vi "flush_trigger_queue.vi"(8 "error in (no error)":errorcluster, 11 "GenericToplevelComponent in":refnum<class "GenericToplevelComponent.lvclass">) -> (0 "error out":errorcluster, 3 "GenericToplevelComponent out":refnum<class "GenericToplevelComponent.lvclass">)   [LabVIEW 2010, in "GenericToplevelComponent.lvclass"]
uses:
  GenericToplevelComponent.lvclass
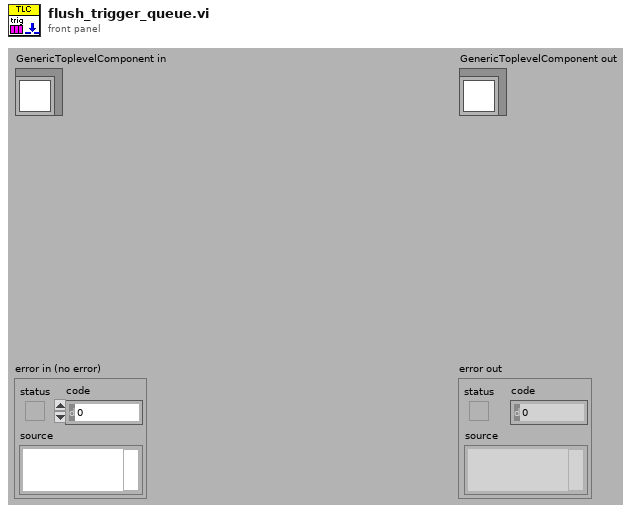
[diagram p1: front panel]
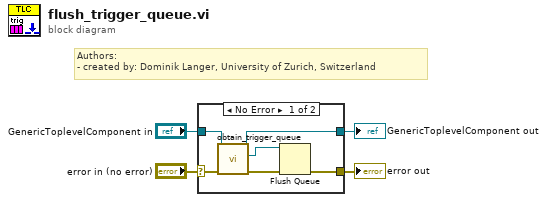
[diagram p0: block diagram]
diagram:
  # "Authors: \n- created by: Dominik Langer, University of Zurich, Switzerland"
  n1 = case shown="No Error" "error in (no error)" {
    selector: "error in (no error)" -> [w10 w12]
    tunnel: [w5 w12] -> w3
    tunnel: [w8 w11] -> w1
    tunnel: "GenericToplevelComponent in" -> [w9 w11]
    frame No Error {
      n2 = call-dynamic "obtain_trigger_queue.vi"("error in (no error)"=w10, "GenericPlugin in"=w9) -> ("error out"=w6:errorcluster, "trigger queue"=w7:refnum<queue>, "GenericPlugin out"=w8:refnum<class "GenericToplevelComponent.lvclass">)  [unwired: 7 in]
      n3 = Flush Queue(queue=w7, error in (no error)=w6) -> (error out=w5:errorcluster)  [unwired: 2 out]
    }
    frame Error {
    }
  }
  "error out" <- w3
  "GenericToplevelComponent out" <- w1
